vi "getChannelArray.vi"(8 "error in (no error)":errorcluster, 11 "StaticOutputEditor.lvclass in":refnum<class "StaticOutputEditor.lvclass">) -> (0 "error out":errorcluster, 2 "ChannelArray":refnum<class "ChannelArray.lvclass">, 3 "StaticOutputEditor.lvclass out":refnum<class "StaticOutputEditor.lvclass">)   [LabVIEW 2009, in "Views.lvlib" / "ScriptEditor.lvlib" / "StaticOutputEditor.lvclass"]
uses:
  StaticOutputEditor.lvclass
  Tools/DatabaseHelpers/Database Objects/ChannelArray/ChannelArray.lvclass
  StaticOutputEditor.lvclass/StaticOutputEditor.ctl
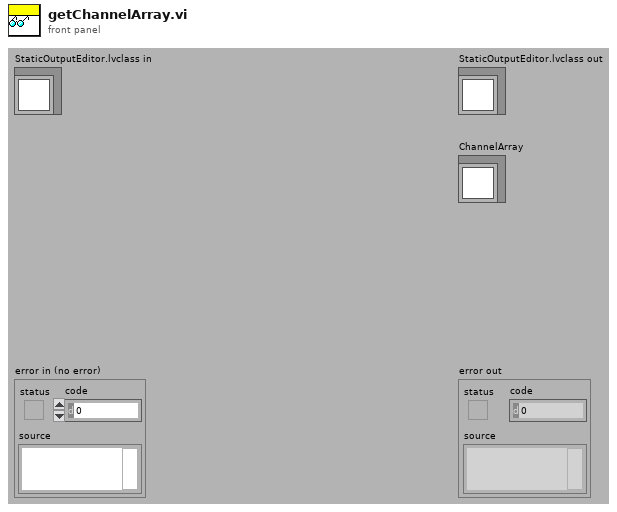
[diagram p1: front panel]
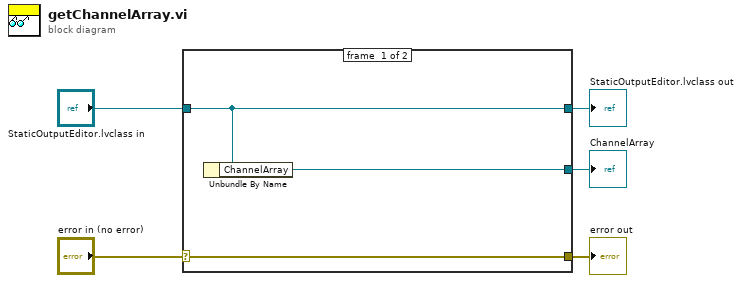
[diagram p0: block diagram]
diagram:
  n1 = case shown="No Error" "error in (no error)" {
    selector: "error in (no error)" -> [w8 w9]
    tunnel: [w8 w9] -> w4
    tunnel: [w7 w10] -> w2
    tunnel: "StaticOutputEditor.lvclass in" -> [w7 w10]
    tunnel: [w6 _] -> w1
    frame #0 {
      n2 = Unbundle By Name(w7) -> ("ChannelArray"=w6:refnum<class "ChannelArray.lvclass">)
    }
    frame #1 {
    }
  }
  "error out" <- w4
  "StaticOutputEditor.lvclass out" <- w2
  "ChannelArray" <- w1
